vi "BuildFilterInput.vi"(10 "Q in":fxp<+/-,16,14>, 11 "I in":fxp<+/-,16,14>) -> (3 "Filter input":fxp<+,32,32>)   [LabVIEW 2013]
uses:
  <vilib>/rvi/FXPMathLib/FxpInterpret/XNode/nifxpmath_Interpret.xnode
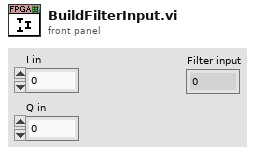
[diagram p1: front panel]
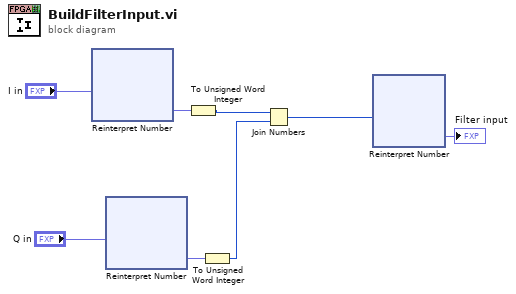
[diagram p0: block diagram]
diagram:
  n1 = xnode "Reinterpret Number"("x"="I in") -> ("y"=w7:fxp<+,16,16>)
  n2 = xnode "Reinterpret Number"("x"="Q in") -> ("y"=w4:fxp<+,16,16>)
  n3 = To Unsigned Word Integer(number=w7) -> (unsigned 16bit integer=w5:u16)
  n4 = To Unsigned Word Integer(number=w4) -> (unsigned 16bit integer=w2:u16)
  n5 = Join Numbers(hi=w5, lo=w2) -> ((hi.lo)=w8:u32)
  n6 = xnode "Reinterpret Number"("x"=w8) -> ("y"=→"Filter input":fxp<+,32,32>)
